vi "Item_Tag_to_Value.vi"(6 "Error in (no error)":errorcluster, 8 "Menu Refnum":refnum<k9>, 9 "Value Mode":string, 10 "Value Source":string, 11 "Item Tag":string) -> (0 "Output Path":path, 1 "Output Boolean":bool, 2 "Output Number":dbl, 3 "Output String":string, 4 "Error out":errorcluster)   [LabVIEW 2013]
uses:
  Global.vi
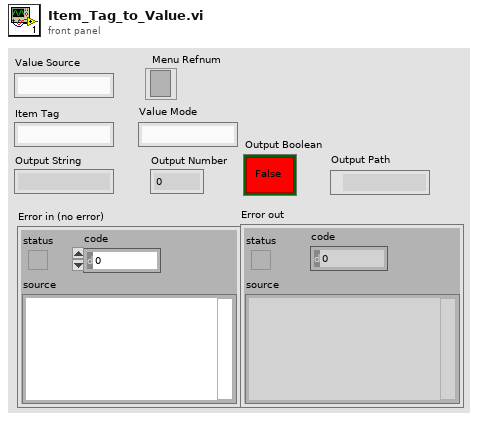
[diagram p1: front panel]
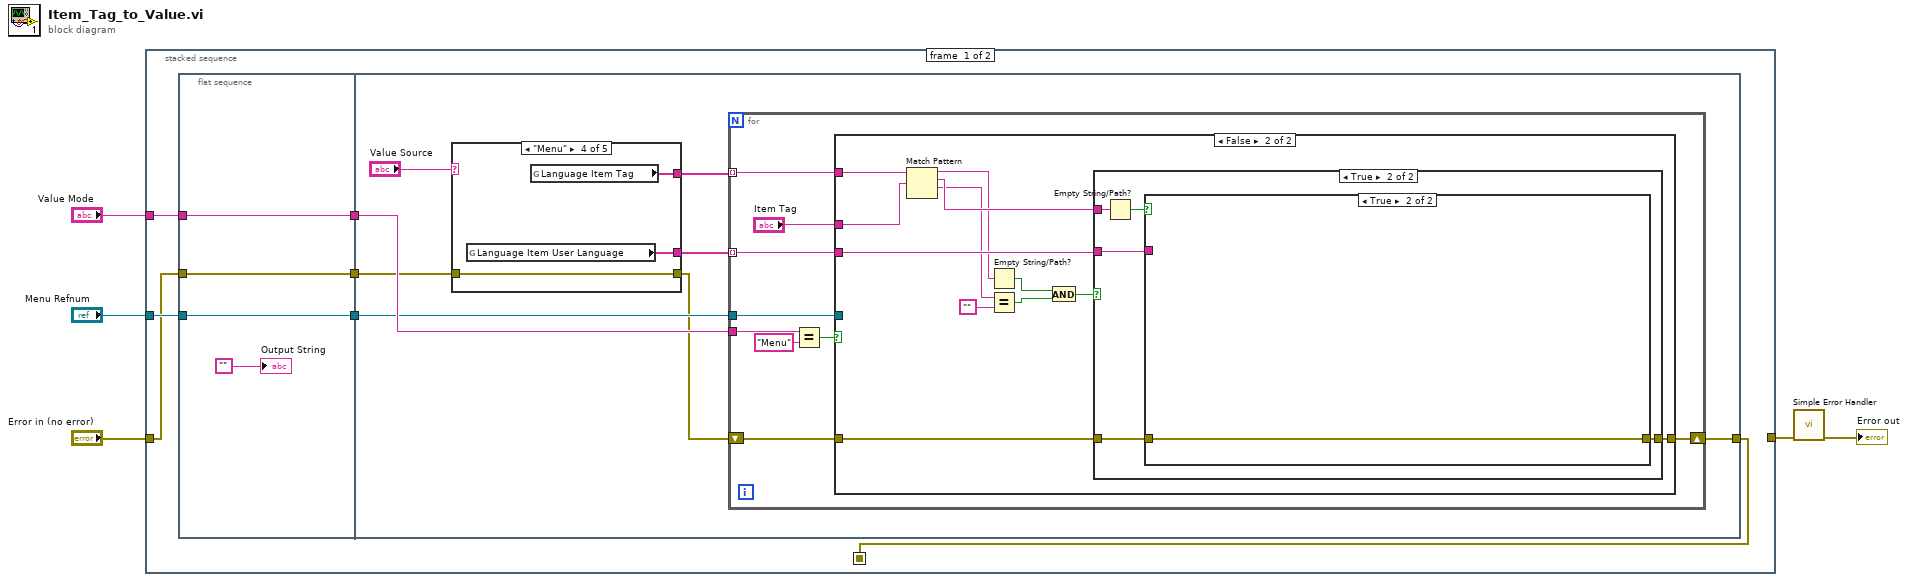
[diagram p0: block diagram]
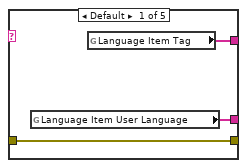
[diagram p2: hidden frame]
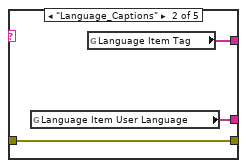
[diagram p3: hidden frame]
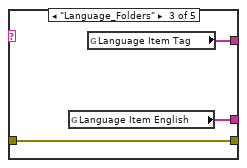
[diagram p4: hidden frame]
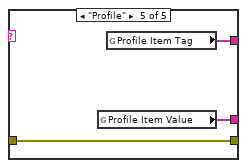
[diagram p5: hidden frame]
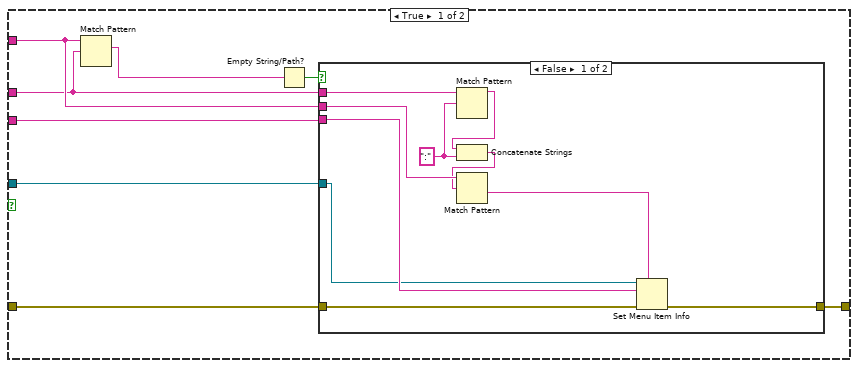
[diagram p6: hidden frame]
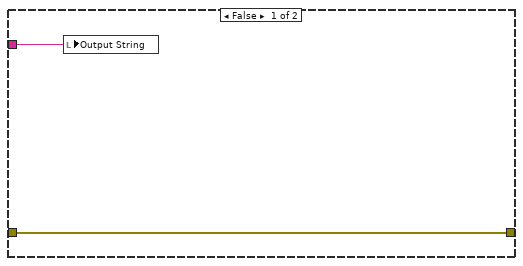
[diagram p9: hidden frame]
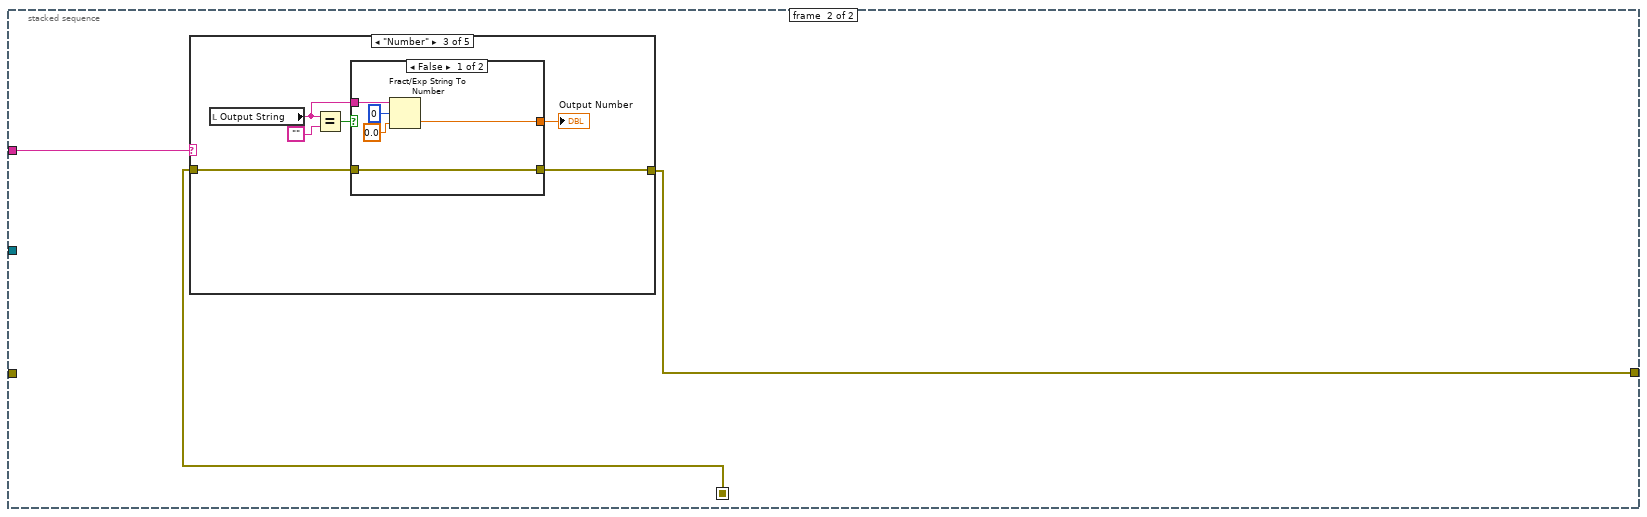
[diagram p10: hidden frame]
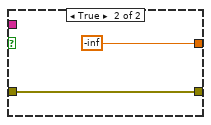
[diagram p13: hidden frame]
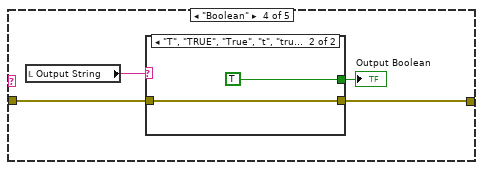
[diagram p14: hidden frame]
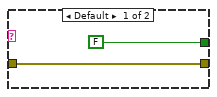
[diagram p15: hidden frame]
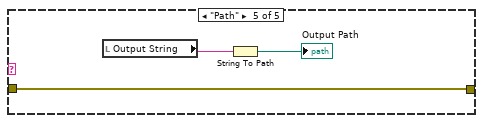
[diagram p16: hidden frame]
diagram:
  n1 = stacked-sequence {
    seq-local: [w10 _] -> [_ w90]
    tunnel: "Value Mode" -> [w12 w91]
    tunnel: "Menu Refnum" -> [w11 _]
    tunnel: "Error in (no error)" -> [w9 _]
    tunnel: [_ w89] -> w2
    frame #0 {
      n2 = flat-sequence {
        tunnel: w9 -> [w14]
        tunnel: w11 -> [w15]
        tunnel: w12 -> [w16]
        tunnel: [w16] -> w8
        tunnel: [w15] -> w7
        tunnel: [w14] -> w6
        tunnel: [w19] -> w10
        tunnel: w8 -> [w21]
        tunnel: w7 -> [w20]
        tunnel: w6 -> [w18]
        frame #0 {
          "Output String" <- ""
        }
        frame #1 {
          n3 = case shown="\"Menu\"" "Value Source" {
            tunnel: [w27 w30 w33 w36 w39] -> w22
            tunnel: [w26 w29 w32 w35 w38] -> w23
            tunnel: w18 -> [w25 w28 w31 w34 w37]
            tunnel: [w25 w28 w31 w34 w37] -> w17
            frame Default {
              n4 = global read "Global.vi" "Language Item User Language"() -> (w26:string[])
              n5 = global read "Global.vi" "Language Item Tag"() -> (w27:string[])
            }
            frame "Language_Captions" {
              n6 = global read "Global.vi" "Language Item User Language"() -> (w29:string[])
              n7 = global read "Global.vi" "Language Item Tag"() -> (w30:string[])
            }
            frame "Language_Folders" {
              n8 = global read "Global.vi" "Language Item English"() -> (w32:string[])
              n9 = global read "Global.vi" "Language Item Tag"() -> (w33:string[])
            }
            frame "Menu" {
              n10 = global read "Global.vi" "Language Item User Language"() -> (w35:string[])
              n11 = global read "Global.vi" "Language Item Tag"() -> (w36:string[])
            }
            frame "Profile" {
              n12 = global read "Global.vi" "Profile Item Value"() -> (w38:string[])
              n13 = global read "Global.vi" "Profile Item Tag"() -> (w39:string[])
            }
          }
          n14 = for {
            tunnel: w22 -> [w47] mode=indexing
            tunnel: w23 -> [w48] mode=indexing
            tunnel: w21 -> [w43]
            tunnel: w20 -> [w46]
            shift-right: [w40] -> w19
            shift-left: w17 -> [w41]
            n15 = Equal?(x=w43, y="Menu") -> (x = y?=w42:bool)
            n16 = case shown="False" w42 {
              tunnel: w48 -> [w56 w79]
              tunnel: w47 -> [w54 w76]
              tunnel: w46 -> [w53 _]
              tunnel: "Item Tag" -> [w52 w70]
              tunnel: w41 -> [w50 w69]
              tunnel: [w49 w68] -> w40
              frame True {
                n17 = Match Pattern(string=w54, regular expression=w52) -> (match substring=w55:string)  [unwired: 1 in, 3 out]
                n18 = Empty String/Path?(string/path=w55) -> (empty?=w51:bool)
                n19 = case shown="False" w51 {
                  tunnel: w56 -> [w66 _]
                  tunnel: w54 -> [w65 _]
                  tunnel: w53 -> [w64 _]
                  tunnel: w52 -> [w63 _]
                  tunnel: w50 -> [w58 w67]
                  tunnel: [w57 w67] -> w49
                  frame False {
                    w61 = ":" ("regular expression")
                    n20 = Match Pattern(string=w63, regular expression=w61) -> (before substring=w62:string)  [unwired: 1 in, 3 out]
                    n21 = Concatenate Strings(w62, w61) -> (w60:string)
                    n22 = Match Pattern(string=w65, regular expression=w60) -> (after substring=w59:string)  [unwired: 1 in, 3 out]
                    n23 = Set Menu Item Info(7:w59, 8:w58, 10:w66, 11:w64) -> (0:w57:errorcluster)  [unwired: 3 in, 1 out]
                  }
                  frame True {
                  }
                }
              }
              frame False {
                n24 = Match Pattern(string=w76, regular expression=w70) -> (before substring=w77:string, match substring=w78:string, after substring=w72:string)  [unwired: 1 in, 1 out]
                n25 = Empty String/Path?(string/path=w77) -> (empty?=w74:bool)
                n26 = Equal?(x=w72, y="") -> (x = y?=w73:bool)
                n27 = And(x=w74, y=w73) -> (x .and. y?=w75:bool)
                n28 = case shown="True" w75 {
                  tunnel: w79 -> [_ w84]
                  tunnel: w78 -> [_ w83]
                  tunnel: w69 -> [w80 w82]
                  tunnel: [w80 w81] -> w68
                  frame False {
                  }
                  frame True {
                    n29 = Empty String/Path?(string/path=w83) -> (empty?=w85:bool)
                    n30 = case shown="True" w85 {
                      tunnel: w84 -> [w87 _]
                      tunnel: w82 -> [w86 w88]
                      tunnel: [w86 w88] -> w81
                      frame False {
                        n31 = local write "Output String"(w87) -> ()
                      }
                      frame True {
                      }
                    }
                  }
                }
              }
            }
          }
        }
      }
    }
    frame #1 {
      n32 = case shown="\"Number\"" w91 {
        tunnel: w90 -> [w92 w93 w96 w109 w116]
        tunnel: [w92 w93 w95 w108 w116] -> w89
        frame "String", Default {
          # "No action required"
        }
        frame "Menu" {
          # "No action required"
        }
        frame "Number" {
          n33 = local read "Output String"() -> (w97:string)
          n34 = Equal?(x=w97, y="") -> (x = y?=w99:bool)
          n35 = case shown="False" w99 {
            tunnel: w97 -> [w102 _]
            tunnel: w96 -> [w101 w106]
            tunnel: [w101 w106] -> w95
            tunnel: [w100 -inf] -> w94
            frame False {
              n36 = Fract/Exp String To Number(string=w102, offset=0, default (0 dbl)=0.0 ("default (0 I32)")) -> (number=w100:dbl)  [unwired: 1 in, 1 out]
            }
            frame True {
            }
          }
          "Output Number" <- w94
        }
        frame "Boolean" {
          n37 = local read "Output String"() -> (w110:string)
          n38 = case shown="\"T\", \"TRUE\", \"True\", \"t\", \"true\"" w110 {
            tunnel: w109 -> [w112 w113]
            tunnel: [w112 w113] -> w108
            tunnel: [FALSE ("Output Boolean") TRUE] -> w107
            frame Default {
            }
            frame "T", "TRUE", "True", "t", "true" {
            }
          }
          "Output Boolean" <- w107
        }
        frame "Path" {
          n39 = local read "Output String"() -> (w117:string)
          n40 = String To Path(string=w117) -> (path=→"Output Path":path)
        }
      }
    }
  }
  n41 = call <vilib>:"Simple Error Handler.vi"("error in (no error)"=w2) -> ("error out"=→"Error out":errorcluster)  [unwired: 4 in, 4 out]
